vi "Single Command (No results).vi"(8 "error in (no error)":errorcluster, 9 "Variant (Cluster, Array,..)":variant, 10 "SQL (Single Command)":string, 11 "PQ Connection in":refnum<class "PQ Connection.lvclass">) -> (0 "error out":errorcluster, 3 "PQ Connection out":refnum<class "PQ Connection.lvclass">)   [LabVIEW 2015, in "PQ Connection.lvclass"]
uses:
  PQ Connection.lvclass
  Result/PQ Result.lvclass
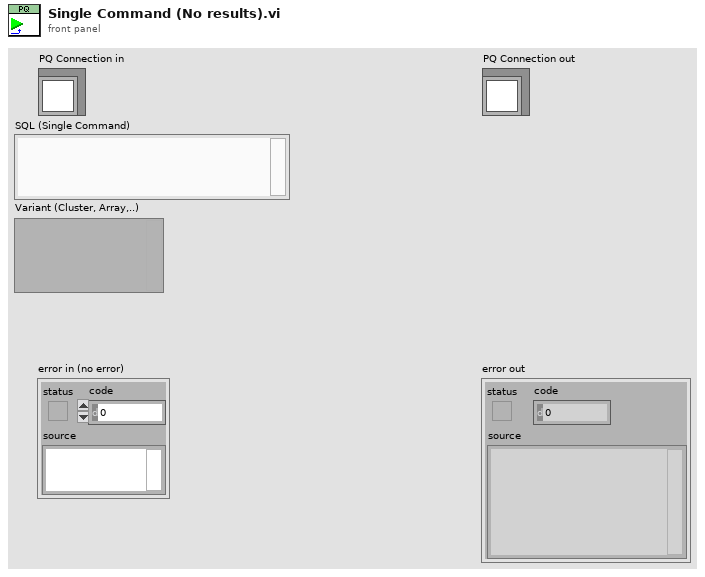
[diagram p1: front panel]
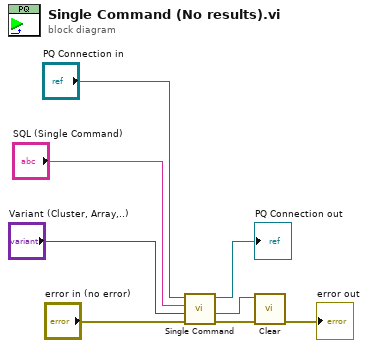
[diagram p0: block diagram]
diagram:
  n1 = call "Single Command.vi"("error in (no error)"="error in (no error)", "Variant (Cluster, Array,..)"="Variant (Cluster, Array,..)", "SQL (Single Command)"="SQL (Single Command)", "PQ Connection in"="PQ Connection in") -> ("error out"=w4:errorcluster, "First Result with Rows returned"=w6:refnum<class "PQ Result.lvclass">, "PQ Connection out"=→"PQ Connection out":refnum<class "PQ Connection.lvclass">)  [unwired: 4 in, 1 out]
  n2 = call "Clear.vi"("error in (no error)"=w4, "PQ Result  in"=w6) -> ("error out"=→"error out":errorcluster)  [unwired: 9 in]
